vi "SetSpriteImage.vi"(7 "SpriteIndex":u8, 8 "error in (no error)":errorcluster, 9 "TransparentColor":fxp<+,3,3>, 10 "ImagePath":path, 11 "Array in":refnum<class "RT_Sprite.lvclass">[](array[class])) -> (0 "error out":errorcluster, 3 "Array out":refnum<class "RT_Sprite.lvclass">[](array[class]))   [LabVIEW 2019, in "RT_Game.lvlib" / "Game.lvclass"]
uses:
  Game.lvclass
  RT_Sprite/RT_Sprite.lvclass
  C:/Users/FreshBob/Dropbox/VIs/myRIO_GameConsole/RT/RT_Game/GameObject/GameObject.lvclass
  GameObject/GameObject.lvclass/GameObject.ctl
  GameObject/Write IsActive.vi
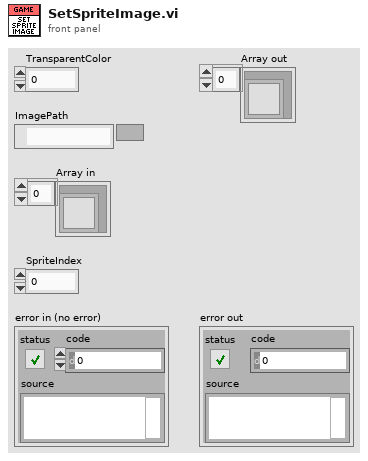
[diagram p1: front panel]
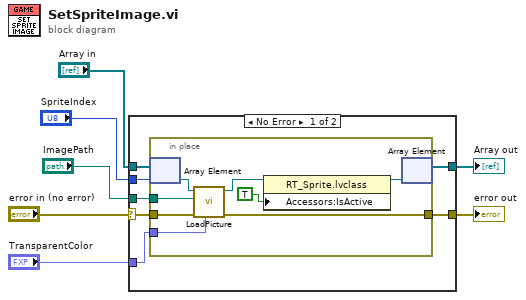
[diagram p0: block diagram]
diagram:
  n1 = case shown="No Error" "error in (no error)" {
    selector: "error in (no error)" -> [w13 w24]
    tunnel: [w12 w24] -> w1
    tunnel: "SpriteIndex" -> [w14 _]
    tunnel: "ImagePath" -> [w11 _]
    tunnel: "TransparentColor" -> [w10 _]
    tunnel: "Array in" -> [w9 w23]
    tunnel: [w8 w23] -> w7
    frame No Error {
      n2 = in-place {
        in-place-border: w13 -> [w22]
        in-place-border: [w21] -> w12
        in-place-border: w11 -> [w18]
        in-place-border: w10 -> [w17]
        n3 = in-place-array #1(w9, w14) -> (w20:refnum<class "RT_Sprite.lvclass">)
        n4 = call "LoadPicture.vi"("Transparent Color"=w17, "error in (no error)"=w22, "Picture Path"=w18, "RT_Sprite in"=w20) -> ("error out"=w21:errorcluster, "RT_Sprite out"=w19:refnum<class "RT_Sprite.lvclass">)  [unwired: 6 in]
        n5 = property class="RT_Sprite.lvclass"(reference=w19, "Accessors:IsActive"=TRUE ("IsActive")) -> (reference out=w16:refnum<class "RT_Sprite.lvclass">)  [unwired: 1 in, 1 out]
        n6 = in-place-array #1(w16) -> (w8:refnum<class "RT_Sprite.lvclass">[])  [unwired: 1 out]
      }
    }
    frame Error {
    }
  }
  "Array out" <- w7
  "error out" <- w1
